vi "Generate LV Icon User Layers.vi"(8 "error in (no error)":errorcluster, 10 "User layers":T1[](array[typedef]), 11 "Icon in":refnum<class "Icon.lvclass">) -> (0 "error out":errorcluster, 3 "Icon out":refnum<class "Icon.lvclass">)   [LabVIEW 2020, in "LabVIEW Icon API.lvlib"]
doc: "Generate LV Icon User Layers overwrites all existing User Layers in the Icon class."
uses:
  LabVIEW Icon API.lvlib
  lv_icon/Controls/Layer.ctl
  lv_icon/Controls/LayerType.ctl
  lv_icon/Classes/Layer/Layer.lvclass
  lv_icon/Classes/Icon/Icon.lvclass
  <vilib>/picture/picture.llb/imagedata.ctl
  API_User Layer Data.ctl
  <vilib>/Utility/miscctls.llb/LVPoint32TypeDef.ctl
panel:
  # "`"
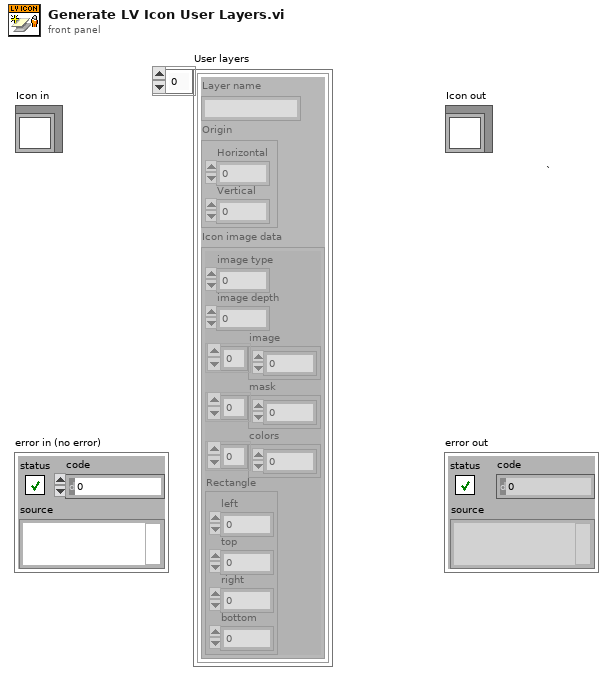
[diagram p1: front panel]
types:
  T1 = typedef "LabVIEW Icon API.lvlib/API_User Layer Data.ctl" = cluster{"Layer name":string, "Origin":T2, "Icon image data":T3}
  T2 = typedef "LVPoint32TypeDef.ctl" = cluster{"Horizontal":i32, "Vertical":i32}
  T3 = typedef "imagedata.ctl" = cluster{"image type":i32, "image depth":i32, "image":u8[], "mask":u8[], "colors":u32[], "Rectangle":cluster{"left":i16, "top":i16, "right":i16, "bottom":i16}}
  T4 = typedef "Layer.ctl" = cluster{"LayerIcon":picture, "LayerName":string, "Opacity":u8, "Visibility?":bool}
  T5 = typedef "LayerType.ctl" = enum16{"Graphic", "Text", "Tool", "Graphic Drop"}
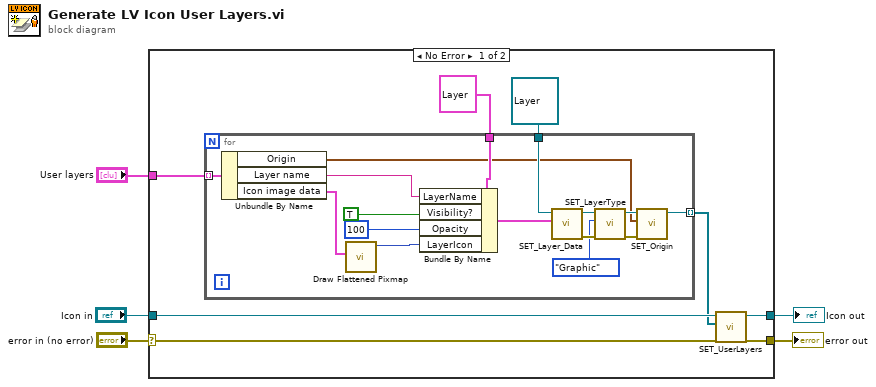
[diagram p0: block diagram]
diagram:
  n1 = case shown="No Error" "error in (no error)" {
    selector: "error in (no error)" -> [w13 w31]
    tunnel: [w12 w31] -> w4
    tunnel: "Icon in" -> [w11 w30]
    tunnel: [w10 w30] -> w2
    tunnel: "User layers" -> [w9 _]
    frame No Error {
      n2 = for {
        tunnel: w9 -> [w29] mode=indexing
        tunnel: T4 {"LayerIcon"=bytes[0], "LayerName"="", "Opacity"=0, "Visibility?"=FALSE} ("Data") -> [w21]
        tunnel: refnum<class "Layer.lvclass"> refnum ("Layer.lvclass in") -> [w20]
        tunnel: [w16] -> w6 mode=indexing
        n3 = Unbundle By Name(w29) -> ("Origin"=w18:T2, "Layer name"=w22:string, "Icon image data"=w15:T3)
        n4 = call <vilib>:"Draw Flattened Pixmap.vi"("image data"=w15) -> ("new picture"=w14:picture)  [unwired: 8 in]
        n5 = Bundle By Name(cluster=w21, "LayerName"=w22, "Visibility?"=TRUE, "Opacity"=u8 100, "LayerIcon"=w14) -> (w25:T4)
        n6 = call-dynamic "SET_Layer_Data.vi"("Data"=w25, "Layer.lvclass in"=w20) -> ("error out"=w26:errorcluster, "Layer.lvclass out"=w24:refnum<class "Layer.lvclass">)  [unwired: 2 in, 6 out]
        n7 = call-dynamic "SET_LayerType.vi"("error in (no error)"=w26, "Type"=LayerType."Graphic", "Layer.lvclass in"=w24) -> ("error out"=w17:errorcluster, "Layer.lvclass out"=w19:refnum<class "Layer.lvclass">)  [unwired: 7 out]
        n8 = call-dynamic "SET_Origin.vi"("error in"=w17, "Point32"=w18, "Layer.lvclass in"=w19) -> ("Layer.lvclass out"=w16:refnum<class "Layer.lvclass">)  [unwired: 7 in, 1 out]
      }
      n9 = call-dynamic "SET_UserLayers.vi"("error in (no error)"=w13, "Layers"=w6, "Icon.lvclass in"=w11) -> ("error out"=w12:errorcluster, "Icon.lvclass out"=w10:refnum<class "Icon.lvclass">)  [unwired: 7 in]
    }
    frame Error {
    }
  }
  "error out" <- w4
  "Icon out" <- w2
